vi "绝对时间与相对时间的加减运算（利用单位）.vi"() -> ()   [LabVIEW 2012]
panel:
  out "之前时间":timestamp
  out "之后时间":timestamp
  in  "时间差（小时）":dbl
  in  "输入时间":timestamp
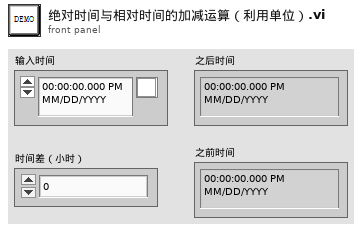
[diagram p1: front panel]
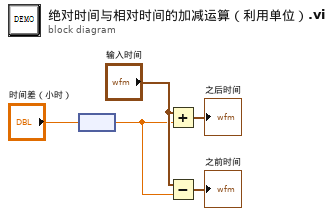
[diagram p0: block diagram]
diagram:
  n1 = node("时间差（小时）") -> (w2:dbl[unit])
  n2 = Add(x="输入时间", y=w2) -> (x+y=→"之后时间":timestamp)
  n3 = Subtract(x="输入时间", y=w2) -> (x-y=→"之前时间":timestamp)
